vi "Create Child Page.vi"(8 "error in (no error)":errorcluster {"code" format="Error %.0f"}, 9 "Parent Page Title":string, 10 "New Page Title":string, 11 "VIDoc Printer - Confluence In":refnum<class "VIDoc Printer - Confluence.lvclass">) -> (0 "error out":errorcluster {"code" format="Error %.0f"}, 1 "Created Page Info":T1, 3 "VIDoc Printer - Confluence Out":refnum<class "VIDoc Printer - Confluence.lvclass">)   [LabVIEW 2023, in "VIDoc Printer - Confluence.lvlib" / "VIDoc Printer - Confluence.lvclass"]
uses:
  VIDoc Printer - Confluence.lvclass
  Types/Page Info.ctl
  <userlib>/_PetranWay/LabVIEW Confluence API/Source/Confluence/Page/Page.lvclass
  VIDoc Printer - Confluence.lvclass/VIDoc Printer - Confluence.ctl
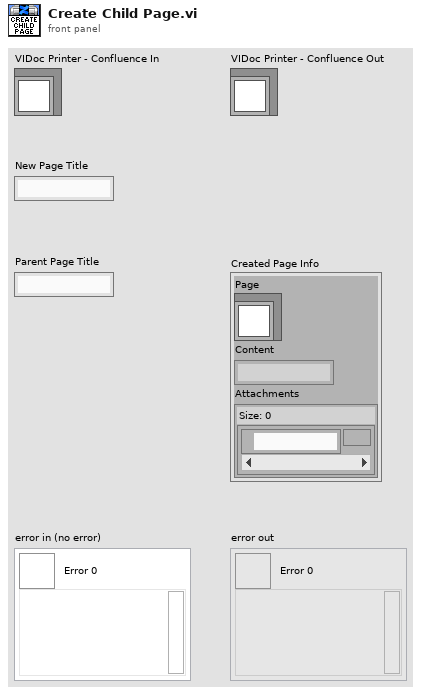
[diagram p1: front panel]
types:
  T1 = typedef "VIDoc Printer - Confluence.lvlib/VIDoc Printer - Confluence.lvclass/Page Info.ctl" = cluster{"Page":refnum<class "Page.lvclass">, "Content":string, "Attachments":set{path}}
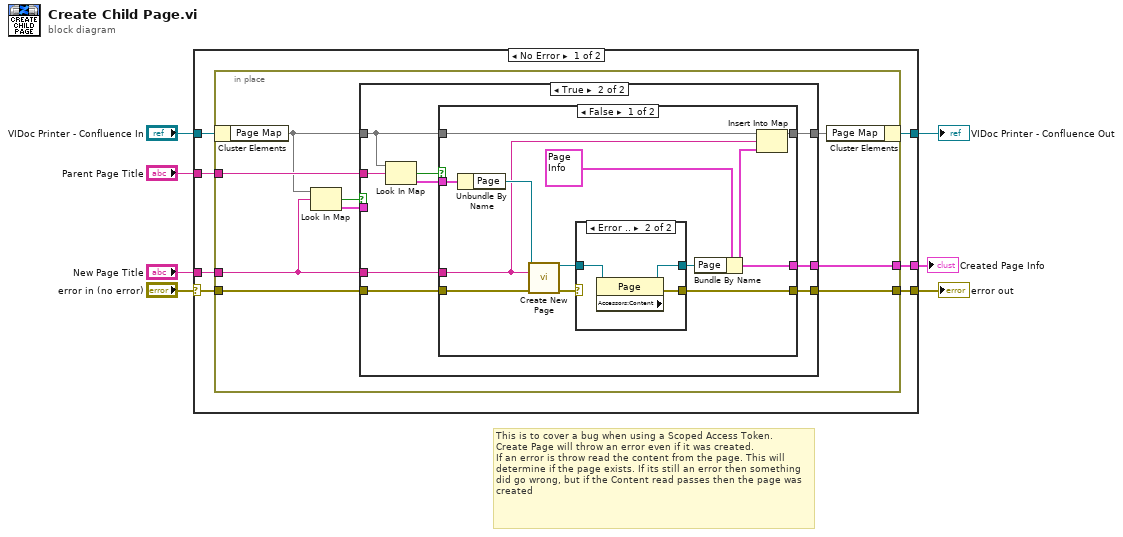
[diagram p0: block diagram]
diagram:
  # "This is to cover a bug when using a Scoped Access Token.\nCreate Page will throw an error even if it was created. \nIf an error is throw read the content from the page. This will determine if the page exists. If its still an error then something did go wrong, but if the Content read passes then the page was created"
  n1 = case shown="No Error" "error in (no error)" {
    selector: "error in (no error)" -> [w12 w56]
    tunnel: [w11 w56] -> w6
    tunnel: [w9 w55] -> w4
    tunnel: "VIDoc Printer - Confluence In" -> [w14 w55]
    tunnel: "Parent Page Title" -> [w13 _]
    tunnel: "New Page Title" -> [w10 _]
    tunnel: [w8 _] -> w1
    frame No Error {
      n2 = in-place {
        in-place-border: w13 -> [w23]
        in-place-border: w12 -> [w22]
        in-place-border: [w21] -> w11
        in-place-border: w10 -> [w18]
        in-place-border: [w16] -> w8
        n3 = in-place-cluster #1(w14) -> ("Page Map"=w19:map{string, T1})
        n4 = Look In Map(map=w19, key=w18) -> (key not found?=w17:bool, value=w15:T1)  [unwired: 1 in]
        n5 = case shown="True" w17 {
          tunnel: w23 -> [_ w35]
          tunnel: w22 -> [w24 w33]
          tunnel: [w24 w32] -> w21
          tunnel: [w25 w30] -> w20
          tunnel: w19 -> [w25 w29]
          tunnel: w18 -> [_ w28]
          tunnel: [w26 w27] -> w16
          tunnel: w15 -> [w26 _]
          frame False {
            # "New Page already exists"
          }
          frame True {
            n6 = Look In Map(map=w29, key=w35) -> (key not found?=w31:bool, value=w34:T1)  [unwired: 1 in]
            n7 = case shown="False" w31 {
              tunnel: w34 -> [w43 _]
              tunnel: w33 -> [w47 w53]
              tunnel: [w36 w53] -> w32
              tunnel: w28 -> [w39 _]
              tunnel: w29 -> [w46 w54]
              tunnel: [w45 w54] -> w30
              tunnel: [w40 _] -> w27
              frame False {
                n8 = Unbundle By Name(w43) -> ("Page"=w42:refnum<class "Page.lvclass">)
                n9 = call-dynamic "Create New Page.vi"("Desired Parent Page"=w42, "New Page Title"=w39, "error in (no error)"=w47) -> ("Created Page"=w41:refnum<class "Page.lvclass">, "error out"=w37:errorcluster)  [unwired: 11 in]
                n10 = case shown="Error .." w37 {
                  selector: w37 -> [w49 _]
                  tunnel: w41 -> [w48 w52]
                  tunnel: [w48 w51] -> w38
                  tunnel: [w49 w50] -> w36
                  frame No Error {
                  }
                  frame Error {
                    n11 = property class="Page" props=["Accessors:Content"](reference=w52) -> (reference out=w51:refnum<class "Page.lvclass">, error out=w50:errorcluster)  [unwired: 1 in, 1 out]
                  }
                }
                n12 = Bundle By Name(cluster=T1 {"Page"=refnum, "Content"="", "Attachments"={}} ("Page Info"), "Page"=w38) -> (w40:T1)
                n13 = Insert Into Map(map in=w46, key=w39, value=w40) -> (map out=w45:map{string, T1})  [unwired: 2 out]
              }
              frame True {
                # "Parent page doesn't exist"
              }
            }
          }
        }
        n14 = in-place-cluster #1("Page Map"=w20) -> (w9:refnum<class "VIDoc Printer - Confluence.lvclass">)
      }
    }
    frame Error {
    }
  }
  "error out" <- w6
  "VIDoc Printer - Confluence Out" <- w4
  "Created Page Info" <- w1
